vi "PantherLAB_Log - Rename DQMH Module.vi"(9 "New Module Library":path, 10 "Module Info (old)":T1, 11 "Project":refnum<vi>) -> (0 "error out":errorcluster)   [LabVIEW 2016]
doc: "_____\nCreated using DQMH Framework: Event Scripter 7.1.0.1450."
uses:
  <vilib>/Delacor/Delacor QMH/Libraries/_Scripting Support/Module Info--cluster.ctl
  <vilib>/Delacor/Delacor QMH/Libraries/_Scripting Support/Module Type--enum.ctl
  PantherDashboard Scripting Hooks/PantherLAB_Log.lvlib
  <vilib>/Delacor/Delacor QMH/Libraries/_Scripting Support/dqmh_lib_DQMH Scripting Support.lvlib
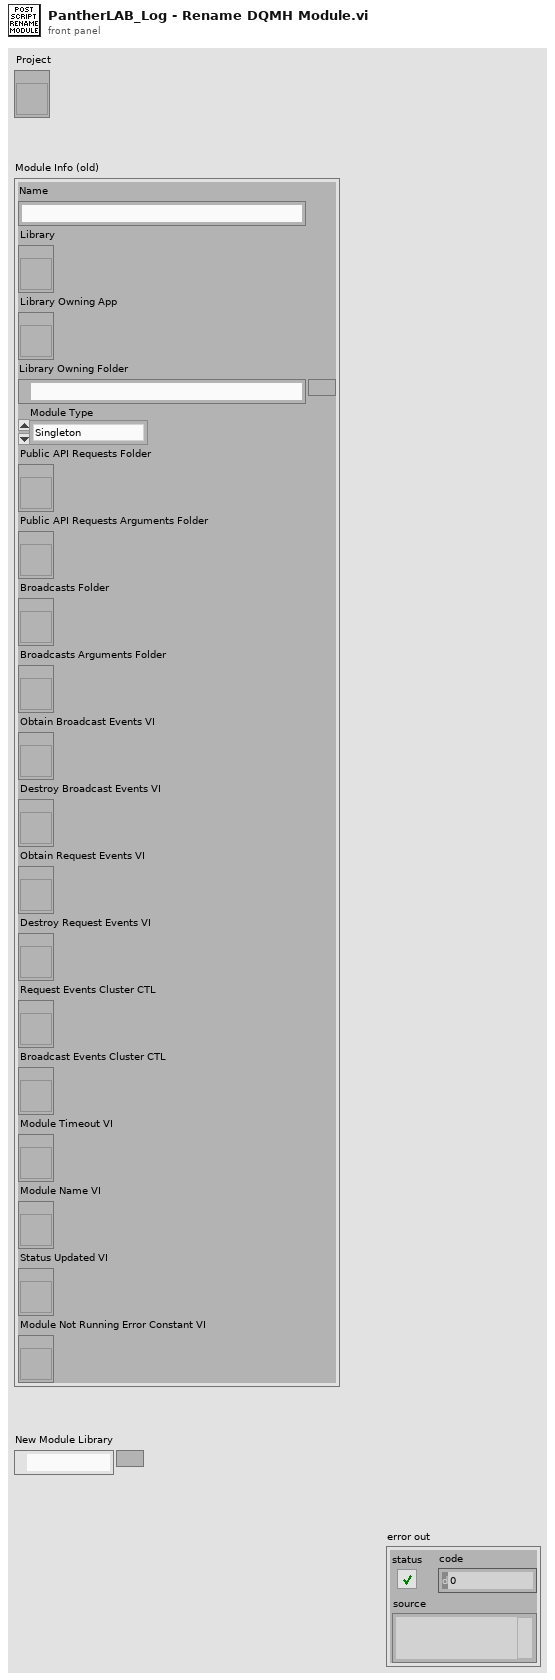
[diagram p1: front panel]
types:
  T1 = typedef "dqmh_lib_DQMH Scripting Support.lvlib/Module Info--cluster.ctl" = cluster{"Name":string, "Library":refnum<vi>, "Library Owning App":refnum<vi>, "Library Owning Folder":path, "Module Type":T2, "Public API Requests Folder":refnum<vi>, "Public API Requests Arguments Folder":refnum<vi>, "Broadcasts Folder":refnum<vi>, "Broadcasts Arguments Folder":refnum<vi>, "Obtain Broadcast Events VI":refnum<vi>, "Destroy Broadcast Events VI":refnum<vi>, "Obtain Request Events VI":refnum<vi>, "Destroy Request Events VI":refnum<vi>, "Request Events Cluster CTL":refnum<vi>, "Broadcast Events Cluster CTL":refnum<vi>, "Module Timeout VI":refnum<vi>, "Module Name VI":refnum<vi>, "Status Updated VI":refnum<vi>, "Module Not Running Error Constant VI":refnum<vi>}
  T2 = typedef "dqmh_lib_DQMH Scripting Support.lvlib/Module Type--enum.ctl" = enum16{"Singleton", "Cloneable"}
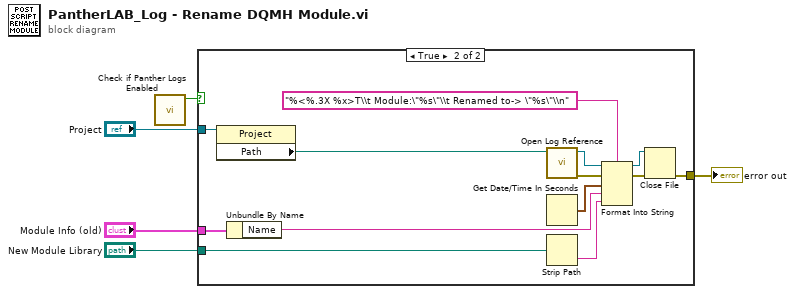
[diagram p0: block diagram]
diagram:
  n1 = call "Check if Panther Logs Enabled.vi"() -> ("PantherLogs Enabled?"=w4:bool)  [unwired: 11 in]
  n2 = case shown="True" w4 {
    tunnel: [_ w16] -> w5
    tunnel: "Project" -> [_ w12]
    tunnel: "Module Info (old)" -> [_ w10]
    tunnel: "New Module Library" -> [_ w9]
    frame False {
    }
    frame True {
      n3 = property class="Project"(reference=w12) -> ("Path"=w11:path)  [unwired: 1 in, 2 out]
      n4 = Unbundle By Name(w10) -> ("Name"=w8:string)
      n5 = call "Open Log Reference.vi"("Project Path"=w11) -> ("error out"=w18:errorcluster, "File Reference"=w15:refnum<file>)  [unwired: 9 in]
      n6 = Get Date/Time In Seconds() -> (seconds since 1Jan1904=w13:timestamp)
      n7 = Strip Path(path=w9) -> (name=w7:string)  [unwired: 1 out]
      n8 = Format Into String(format string="%<%.3X %x>T\\t Module:\"%s\"\\t Renamed to-> \"%s\"\\n", initial string=w15, error in=w18, w13, w8, w7) -> (resulting string=w14:refnum<file>, error out=w17:errorcluster)
      n9 = Close File(refnum=w14, error in=w17) -> (error out=w16:errorcluster)  [unwired: 1 out]
    }
  }
  "error out" <- w5
